vi "MainUI.vi"() -> ()   [LabVIEW 2017]
uses:
  <vilib>/Instr/_visa.llb/VISA Configure Serial Port (Serial Instr).vi
panel:
  in  "MAMP 2":u16
  in  "FCT":u8=24 max=254
  in  "SPM":u16
  in  "Insert":enum32{"OFF", "STOP", "RMPD:1", "RMPD:2"}(radio)
  in  "Delay":dbl
  in  "Insert Delay":bool
  out "Errors":u64
  in  "RES":u8=1 min=1 max=20
  in  "RAMP":u8=2 min=1 max=20
  in  "stop":bool
  in  "VISA resource name":refnum<visa-resource-name>
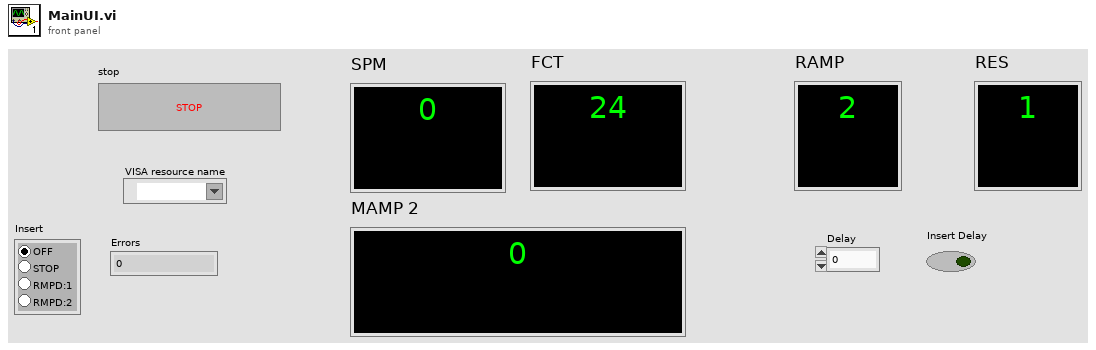
[diagram p1: front panel]
types:
  T1 = enum16{"Init", "Get", "Set Step Counter", "Insert Command"}
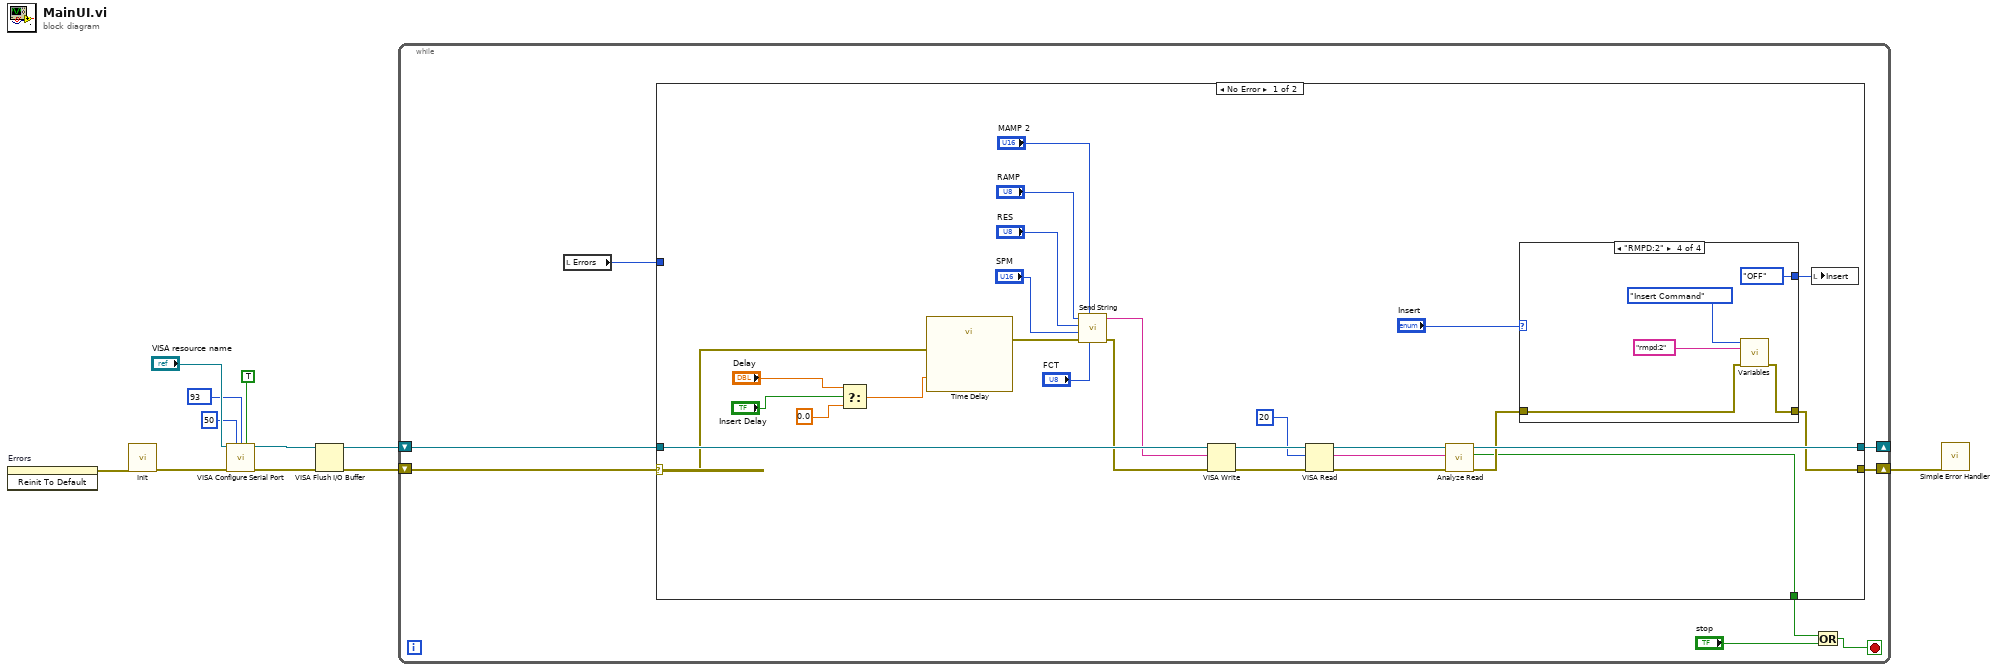
[diagram p0: block diagram]
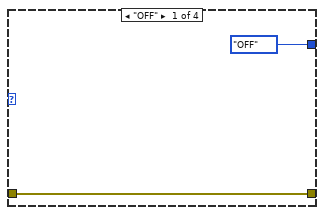
[diagram p2: hidden frame]
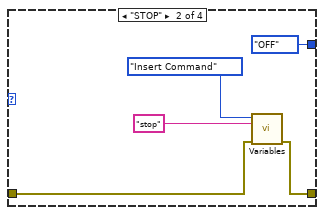
[diagram p3: hidden frame]
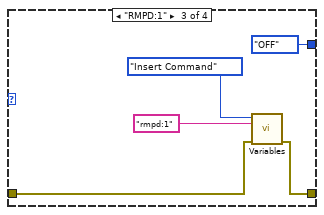
[diagram p4: hidden frame]
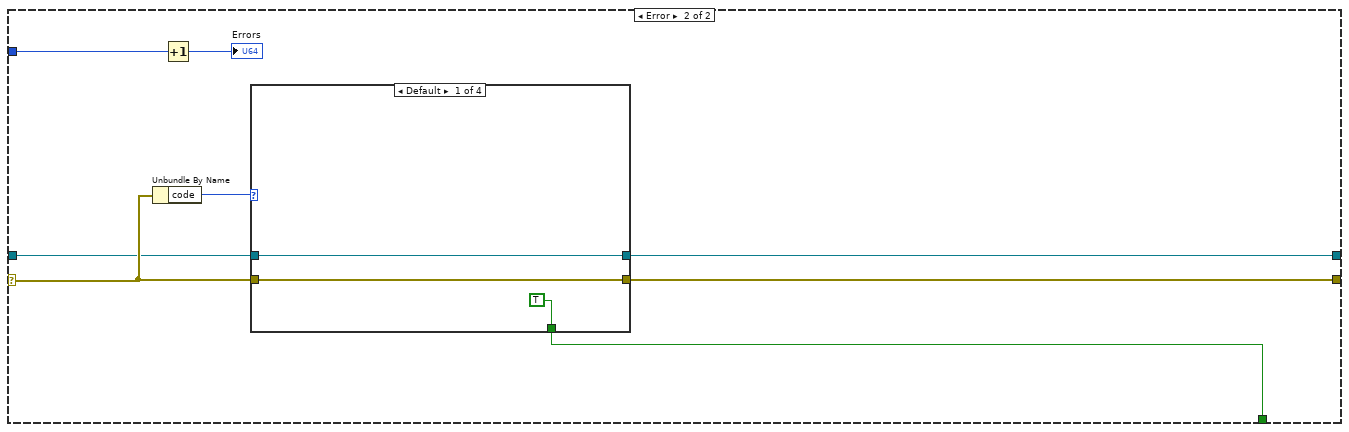
[diagram p5: hidden frame]
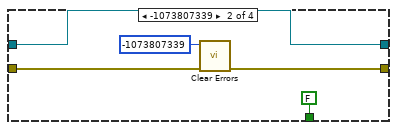
[diagram p6: hidden frame]
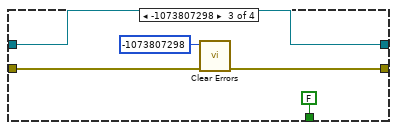
[diagram p7: hidden frame]
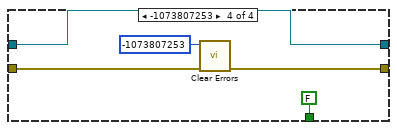
[diagram p8: hidden frame]
diagram:
  n1 = invoke on="Errors" class="DigNum (strict)" method="Reinit To Default"() -> (error out=w1:errorcluster)  [unwired: 3 in, 2 out]
  n2 = call "Init.vi"("error in (no error)"=w1) -> ("error out"=w4:errorcluster)  [unwired: 10 in]
  n3 = call-poly "VISA Configure Serial Port"("VISA resource name"="VISA resource name", "timeout (10sec)"=u32 50, "termination char\n(0xA = '\\n' = LF)"=u8 93 ("termination char\n(0xA = '\\n' = LF)"), "Enable Termination\nChar (T)"=TRUE ("Enable Termination\nChar (T)"), "error in (no error)"=w4) -> ("VISA resource name out"=w8:refnum<visa-resource-name>, "error out"=w7:errorcluster)  [unwired: 9 in]
  n4 = VISA Flush I/O Buffer(VISA resource name=w8, error in (no error)=w7) -> (VISA resource name out=w6:refnum<visa-resource-name>, error out=w5:errorcluster)  [unwired: 1 in]
  n5 = while {
    shift-right: [w19] -> _
    shift-left: w6 -> [w14]
    shift-right: [w18] -> w3
    shift-left: w5 -> [w13]
    stop <- w15 stop-if-true
    n6 = local read "Errors"() -> (w12:u64)
    n7 = case shown="No Error" w13 {
      selector: w13 -> [w29 w69]
      tunnel: w14 -> [w42 w68]
      tunnel: [w36 w67] -> w19
      tunnel: [w32 w66] -> w18
      tunnel: [w31 w65] -> w16
      tunnel: w12 -> [_ w64]
      frame No Error {
        n8 = Select(t="Delay", s="Insert Delay", f=0.0) -> (s? t:f=w27:dbl)
        n9 = call "Time Delay"("error in (no error)"=w29, "Delay Time (s)"=w27) -> ("error out"=w30:errorcluster)  [unwired: 9 in]
        n10 = call "Send String.vi"("FCT"="FCT", "MAMP 2"="MAMP 2", "error in (no error)"=w30, "SPM"="SPM", "RES"="RES", "RAMP"="RAMP") -> ("error out"=w40:errorcluster, "Message"=w41:string)  [unwired: 4 in]
        n11 = VISA Write(VISA resource name=w42, write buffer=w41, error in (no error)=w40) -> (VISA resource name out=w45:refnum<visa-resource-name>, error out=w44:errorcluster)  [unwired: 1 out]
        n12 = VISA Read(VISA resource name=w45, byte count=u32 20, error in (no error)=w44) -> (VISA resource name out=w39:refnum<visa-resource-name>, read buffer=w38:string, error out=w37:errorcluster)  [unwired: 1 out]
        n13 = call "Analyze Read.vi"("VISA in"=w39, "String"=w38, "error in (no error)"=w37) -> ("VISA out"=w36:refnum<visa-resource-name>, "Stop?"=w31:bool, "error out"=w33:errorcluster)  [unwired: 5 in]
        n14 = case shown="\"RMPD:2\"" "Insert" {
          tunnel: w33 -> [w47 w51 w56 w61]
          tunnel: [w47 w50 w55 w60] -> w32
          tunnel: [enum32{"OFF", "STOP", "RMPD:1", "RMPD:2"}."OFF" ("Insert") enum32{"OFF", "STOP", "RMPD:1", "RMPD:2"}."OFF" ("Insert") enum32{"OFF", "STOP", "RMPD:1", "RMPD:2"}."OFF" ("Insert") enum32{"OFF", "STOP", "RMPD:1", "RMPD:2"}."OFF" ("Insert")] -> w23
          frame "OFF" {
          }
          frame "STOP" {
            n15 = call "Variables.vi"("error in (no error)"=w51, "Value"="stop", "Command"=T1."Insert Command") -> ("error out"=w50:errorcluster)  [unwired: 6 in, 2 out]
          }
          frame "RMPD:1" {
            n16 = call "Variables.vi"("error in (no error)"=w56, "Value"="rmpd:1", "Command"=T1."Insert Command") -> ("error out"=w55:errorcluster)  [unwired: 6 in, 2 out]
          }
          frame "RMPD:2" {
            n17 = call "Variables.vi"("error in (no error)"=w61, "Value"="rmpd:2", "Command"=T1."Insert Command") -> ("error out"=w60:errorcluster)  [unwired: 6 in, 2 out]
          }
        }
        n18 = local write "Insert"(w23) -> ()
      }
      frame Error {
        n19 = Unbundle By Name(w69) -> ("code"=w70:i32)
        n20 = Increment(x=w64) -> (x+1=→"Errors":u64)
        n21 = case shown="Default" w70 {
          tunnel: w69 -> [w73 w77 w82 w87]
          tunnel: w68 -> [w72 w75 w80 w85]
          tunnel: [w73 w74 w79 w84] -> w66
          tunnel: [w72 w75 w80 w85] -> w67
          tunnel: [TRUE FALSE FALSE FALSE] -> w65
          frame Default {
          }
          frame -1073807339 {
            n22 = call <vilib>:"Clear Errors.vi"("error in (no error)"=w77, "specific error code to clear (0: all)"=-1073807339) -> ("error out"=w74:errorcluster)  [unwired: 4 in, 1 out]
          }
          frame -1073807298 {
            n23 = call <vilib>:"Clear Errors.vi"("error in (no error)"=w82, "specific error code to clear (0: all)"=-1073807298) -> ("error out"=w79:errorcluster)  [unwired: 4 in, 1 out]
          }
          frame -1073807253 {
            n24 = call <vilib>:"Clear Errors.vi"("error in (no error)"=w87, "specific error code to clear (0: all)"=-1073807253) -> ("error out"=w84:errorcluster)  [unwired: 4 in, 1 out]
          }
        }
      }
    }
    n25 = Or(x=w16, y="stop") -> (x .or. y?=w15:bool)
  }
  n26 = call <vilib>:"Simple Error Handler.vi"("error in (no error)"=w3) -> ()  [unwired: 4 in, 5 out]
